vi "Fixed-Point Configuration.vi"() -> ()   [LabVIEW 2012]
uses:
  Controls/RadixPt.ctl
  <vilib>/Utility/inputDevices.llb/closeMouse.vi
panel:
  out "type string":string="<sign encoding, word length, integer word length>\n<+,8,8>"
  in  "stop":bool
  in  "Signed?":bool
  out "MSB":i32=7
  out "LSB":i32
  out "MSB 8":i32=1
  out "MSB 7":i32=2
  out "MSB 6":i32=3
  out "MSB 5":i32=4
  out "MSB 4":i32=5
  out "MSB 3":i32=6
  in  "Slide":T1=8 scale=-2.0..10.0
  out "Number":dbl=255.0 format="%#_8g"
  in  "0":bool=TRUE
  in  "1":bool=TRUE
  in  "2":bool=TRUE
  in  "3":bool=TRUE
  in  "4":bool=TRUE
  in  "5":bool=TRUE
  in  "6":bool=TRUE
  in  "7":bool=TRUE
  # "="
  # "X"
  # "X"
  # "X"
  # "X"
  # "2"
  # "2"
  # "+"
  # "2"
  # "+"
  # "2"
  # "+"
  # "2"
  # "+"
  # "2"
  # "+"
  # "2"
  # "+"
  # "2"
  # "+"
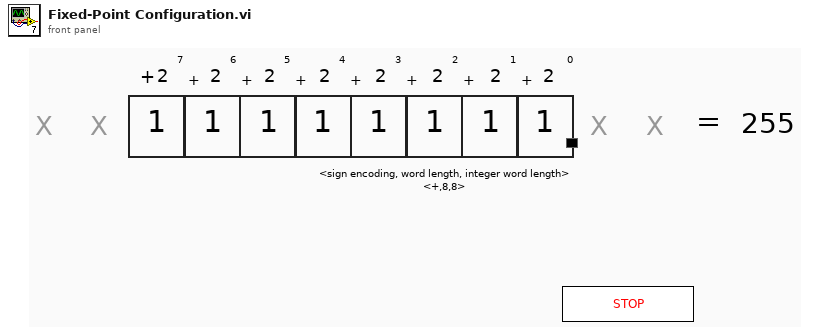
[diagram p1: front panel]
types:
  T1 = typedef "RadixPt.ctl" = i32
  T2 = typedef "LVPoint32TypeDef.ctl" = cluster{"Horizontal":i32, "Vertical":i32}
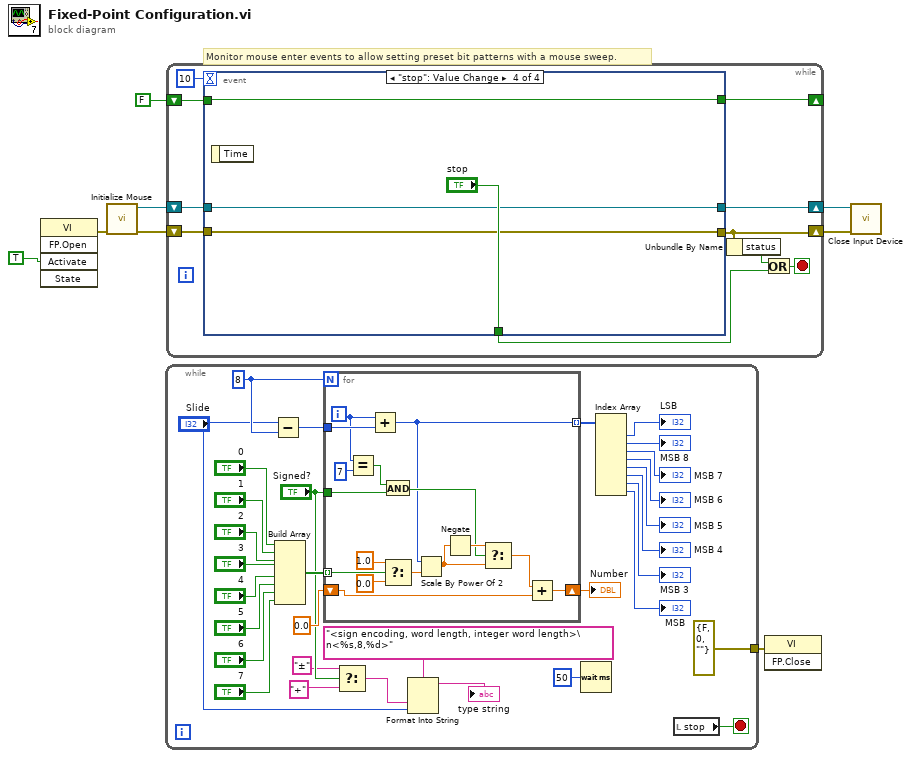
[diagram p0: block diagram]
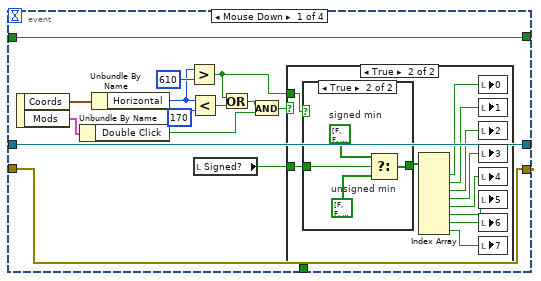
[diagram p2: hidden frame]
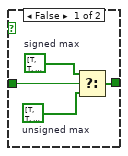
[diagram p4: hidden frame]
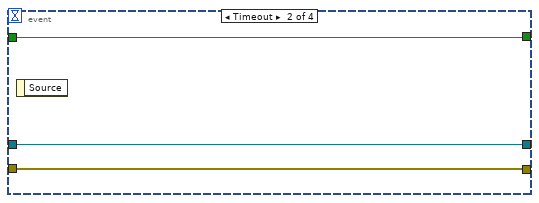
[diagram p5: hidden frame]
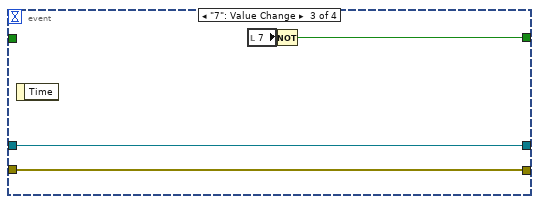
[diagram p6: hidden frame]
diagram:
  # "Monitor mouse enter events to allow setting preset bit patterns with a mouse sweep."
  n1 = invoke class="VI" method="FP.Open"("Activate"=TRUE ("Activate?")) -> (error out=w2:errorcluster)  [unwired: 4 in, 4 out]
  n2 = call <vilib>:"Initialize Mouse.vi"("error in (no error)"=w2) -> ("error out"=w5:errorcluster, "device ID"=w4:refnum<k1>)  [unwired: 9 in]
  n3 = while {
    tunnel: [errorcluster {"status"=FALSE, "code"=0, "source"=""} ("error in (no error)")] -> w8
    stop <- w9 stop-if-true
    w30 = 8 ("y")
    n4 = Subtract(x="Slide", y=w30) -> (x-y=w29:T1)
    n5 = Build Array("0", "1", "2", "3", "4", "5", "6", "7") -> (w33:bool[])
    n6 = for {
      N: w30 -> [_]
      tunnel: w33 -> [w56] mode=indexing
      shift-right: [w51] -> w28
      shift-left: 0.0 ("x") -> [w52]
      tunnel: w29 -> [w50]
      tunnel: [w44] -> w27 mode=indexing
      tunnel: "Signed?" -> [w46]
      i -> [w48]
      n7 = Equal?(x=w48, y=7 ("x")) -> (x = y?=w47:bool)
      n8 = Add(x=w48, y=w50) -> (x+y=w44:T1)
      n9 = And(x=w47, y=w46) -> (x .and. y?=w45:bool)
      n10 = Select(t=1.0 ("x"), s=w56, f=0.0 ("x")) -> (s? t:f=w53:dbl)
      n11 = Scale By Power Of 2(n=w44, x=w53) -> (x*2^n=w43:dbl)
      n12 = Negate(x=w43) -> (-x=w49:dbl)
      n13 = Select(t=w49, s=w45, f=w43) -> (s? t:f=w42:dbl)
      n14 = Add(x=w42, y=w52) -> (x+y=w51:dbl)
    }
    "Number" <- w28
    n15 = Select(t="±", s="Signed?", f="+") -> (s? t:f=w13:string)
    n16 = Format Into String(format string="<sign encoding, word length, integer word length>\n<%s,8,%d>", w13, "Slide") -> (resulting string=→"type string":string)  [unwired: 2 in, 1 out]
    n17 = Wait (ms)(milliseconds to wait=u32 50) -> ()  [unwired: 1 out]
    n18 = Index Array(array=w27) -> (element #1=→"LSB":T1, element #2=→"MSB 8":T1, element #3=→"MSB 7":T1, element #4=→"MSB 6":T1, element #5=→"MSB 5":T1, element #6=→"MSB 4":T1, element #7=→"MSB 3":T1, element #8=→"MSB":T1)  [unwired: 8 in]
    n19 = local read "stop"() -> (w9:bool)
  }
  n20 = while {
    shift-right: [w65] -> _
    shift-left: FALSE ("7") -> [w64]
    shift-right: [w62] -> w6
    shift-left: w5 -> [w63]
    shift-right: [w58] -> w3
    shift-left: w4 -> [w66]
    stop <- w60 stop-if-true
    n21 = event shown="[3] \"stop\": Value Change" {
      selector: _ -> [_ _ _ _]
      dyn-events: _ -> [_ _ _ _]
      timeout: 10 -> [_ _ _ _]
      tunnel: w66 -> [w68 w100 w104 w108]
      tunnel: [w67 w101 w103 w107] -> w65
      tunnel: w64 -> [w67 w101 _ w107]
      tunnel: w63 -> [w69 w102 w105 w109]
      tunnel: [w69 w102 w105 w109] -> w62
      tunnel: [w68 w100 w104 w108] -> w58
      tunnel: [_ _ _ "stop"] -> w57
      event Mouse Down {
        n22 = event-data() -> ("Coords"=w79:T2, "Mods"=w80:cluster{"Double Click":bool, "Menu Key":bool})  [unwired: 1 in]
        n23 = Unbundle By Name(w80) -> ("Double Click"=w78:bool)
        n24 = Unbundle By Name(w79) -> ("Horizontal"=w75:i32)
        n25 = Greater?(x=w75, y=610) -> (0:w71:bool)
        n26 = Less?(x=w75, y=170) -> (x < y?=w74:bool)
        n27 = local read "Signed?"() -> (w70:bool)
        n28 = Or(x=w71, y=w74) -> (x .or. y?=w72:bool)
        n29 = And(x=w72, y=w78) -> (x .and. y?=w73:bool)
        n30 = case shown="True" w73 {
          tunnel: w71 -> [_ w91]
          tunnel: w70 -> [_ w90]
          frame False {
          }
          frame True {
            n31 = case shown="True" w91 {
              tunnel: w90 -> [w95 w99]
              tunnel: [w92 w98] -> w89
              frame False {
                w94 = bool[] [TRUE, TRUE, TRUE, TRUE, TRUE, TRUE, TRUE, FALSE]  # signed max
                w93 = bool[] [TRUE, TRUE, TRUE, TRUE, TRUE, TRUE, TRUE, TRUE]  # unsigned max
                n32 = Select(t=w94, s=w95, f=w93) -> (s? t:f=w92:bool[])
              }
              frame True {
                w97 = bool[] [FALSE, FALSE, FALSE, FALSE, FALSE, FALSE, FALSE, TRUE]  # signed min
                w96 = bool[] [FALSE, FALSE, FALSE, FALSE, FALSE, FALSE, FALSE, FALSE]  # unsigned min
                n33 = Select(t=w97, s=w99, f=w96) -> (s? t:f=w98:bool[])
              }
            }
            n34 = Index Array(array=w89) -> (element #1=w88:bool, element #2=w87:bool, element #3=w86:bool, element #4=w85:bool, element #5=w84:bool, element #6=w83:bool, element #7=w82:bool, element #8=w81:bool)  [unwired: 8 in]
            n35 = local write "0"(w88) -> ()
            n36 = local write "1"(w87) -> ()
            n37 = local write "2"(w86) -> ()
            n38 = local write "3"(w85) -> ()
            n39 = local write "4"(w84) -> ()
            n40 = local write "5"(w83) -> ()
            n41 = local write "6"(w82) -> ()
            n42 = local write "7"(w81) -> ()
          }
        }
      }
      event Timeout {
        n43 = event-data() -> ()  [unwired: 1 in, 1 out]
      }
      event "7": Value Change {
        n44 = event-data() -> ()  [unwired: 1 in, 1 out]
        n45 = local read "7"() -> (w106:bool)
        n46 = Not(x=w106) -> (.not. x?=w103:bool)
      }
      event "stop": Value Change {
        n47 = event-data() -> ()  [unwired: 1 in, 1 out]
      }
    }
    n48 = Unbundle By Name(w62) -> ("status"=w61:bool)
    n49 = Or(x=w61, y=w57) -> (x .or. y?=w60:bool)
  }
  n50 = invoke class="VI" method="FP.Close"(error in=w8) -> ()  [unwired: 2 in, 3 out]
  n51 = call-poly <vilib>:"Close Input Device.vi"("error in (no error)"=w6, "device ID"=w3) -> ()  [unwired: 8 in, 1 out]
